vi "getSocketData.vi"(8 "error in (no error)":errorcluster, 10 "Machine":string, 11 "connection reference":T1) -> (0 "error out":errorcluster, 2 "array":string[][](array[string]), 3 "connection reference 2":T1)   [LabVIEW 2012]
uses:
  <vilib>/addons/database/Connection.llb/Conn ObjectReference.ctl
  <vilib>/addons/database/Connection.llb/Conn Execute.vi
  <vilib>/addons/database/Recordset.llb/Rec Fetch Recordset Data (R).vi
  <vilib>/addons/database/Recordset.llb/Rec Destroy - Connection.vi
  <vilib>/addons/database/_DB Variant To Data/Database Variant To Data.xnode
  <vilib>/addons/database/NI_Database_API.lvlib
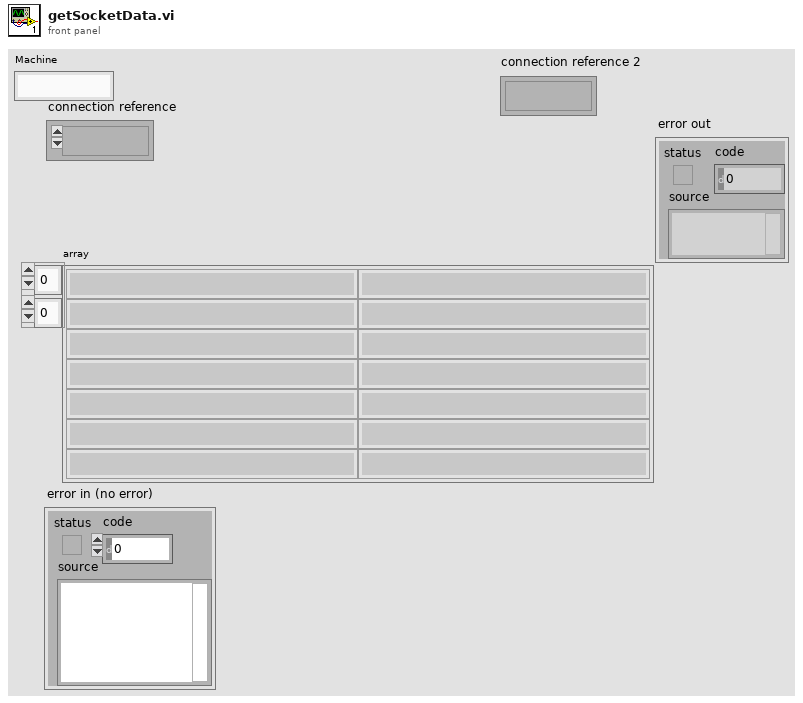
[diagram p1: front panel]
types:
  T1 = typedef "NI_Database_API.lvlib/Conn ObjectReference.ctl" = refnum<k1>
  T2 = typedef "NI_Database_API.lvlib/Rec ObjectReference.ctl" = refnum<k1>
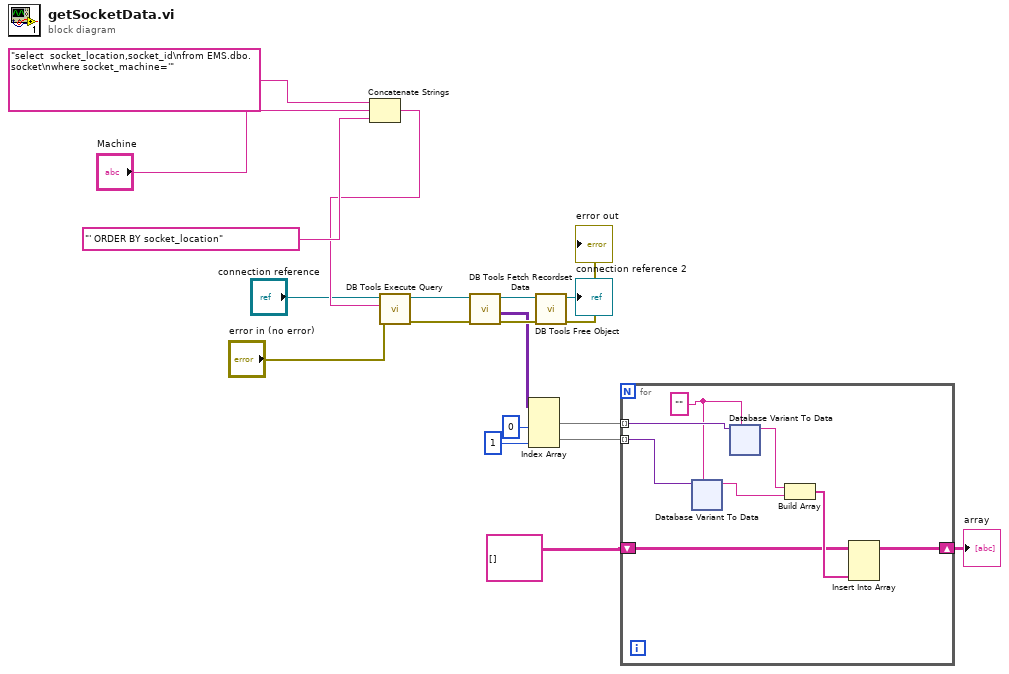
[diagram p0: block diagram]
diagram:
  n1 = Concatenate Strings("select  socket_location,socket_id\nfrom EMS.dbo.socket\nwhere socket_machine='" ("SQL query"), "Machine", "' ORDER BY socket_location" ("string")) -> (w12:string)
  n2 = call-poly <vilib>:"DB Tools Execute Query.vi"("error in (no error)"="error in (no error)", "SQL query"=w12, "connection reference"="connection reference") -> ("error out"=w18:errorcluster, "recordset reference"=w19:T2)  [unwired: 5 in]
  n3 = call-poly <vilib>:"DB Tools Fetch Recordset Data.vi"("error in (no error)"=w18, "recordset reference"=w19) -> ("error out"=w16:errorcluster, "recordset data"=w11:variant[][], "recordset reference out"=w17:T2)  [unwired: 3 in]
  n4 = Index Array(array=w11, index (col) #1=0 ("disabled index (col)"), index (col) #2=1 ("index (col)")) -> (element #1=w8:variant[], element #2=w7:variant[])  [unwired: 2 in]
  n5 = call-poly <vilib>:"DB Tools Free Object.vi"("error in (no error)"=w16, "recordset reference"=w17) -> ("error out"=→"error out":errorcluster, "connection reference"=→"connection reference 2":T1)  [unwired: 8 in]
  n6 = for {
    tunnel: w8 -> [w27] mode=indexing
    tunnel: w7 -> [w26] mode=indexing
    shift-right: [w24] -> w5
    shift-left: string[][] [] ("array") -> [w20]
    w25 = ""
    n7 = xnode "Database Variant To Data"("database variant"=w26, "type"=w25) -> ("data"=w22:string)  [unwired: 1 in, 1 out]
    n8 = xnode "Database Variant To Data"("database variant"=w27, "type"=w25) -> ("data"=w23:string)  [unwired: 1 in, 1 out]
    n9 = Build Array(w23, w22) -> (w21:string[])
    n10 = Insert Into Array(array=w20, new element=w21) -> (w24:string[][])  [unwired: 2 in]
  }
  "array" <- w5
